vi "Close.vi"(0 "VISA Resource Name":refnum<visa-resource-name>, 11 "error in (no error)":errorcluster) -> (15 "error out":errorcluster)   [LabVIEW 2017, in "Agilent 34970.lvlib"]
doc: "This VI closes the I/O interface with the instrument."
uses:
  <instrlib>/Agilent 34970/Agilent 34970.lvlib
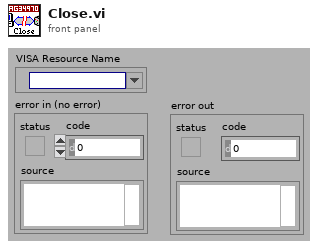
[diagram p1: front panel]
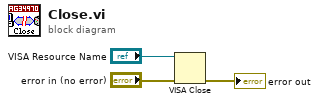
[diagram p0: block diagram]
diagram:
  n1 = VISA Close(VISA resource name="VISA Resource Name", error in (no error)="error in (no error)") -> (error out=→"error out":errorcluster)
